vi "Read Rank.vi"(8 "error in":errorcluster, 11 "SA 26GHz Path Group in":refnum<class "SA 26GHz Path Group.lvclass">) -> (0 "error out":errorcluster, 2 "Rank":dbl, 3 "SA 26GHz Path Group out":refnum<class "SA 26GHz Path Group.lvclass">)   [LabVIEW 2023, in "RFFixtureCharact.PXI.lvlib" / "SA 26GHz Path Group.lvclass"]
uses:
  SA 26GHz Path Group.lvclass
  SA 26GHz Path Group.lvclass/SA 26GHz Path Group.ctl
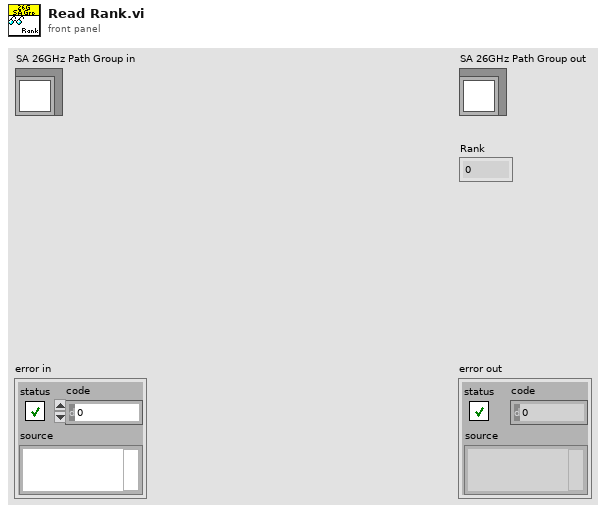
[diagram p1: front panel]
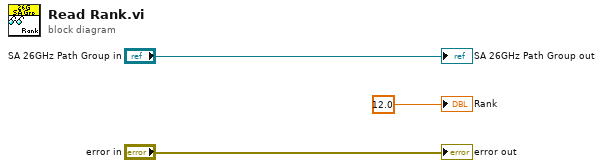
[diagram p0: block diagram]
diagram:
  "error out" <- "error in"
  "SA 26GHz Path Group out" <- "SA 26GHz Path Group in"
  "Rank" <- 12.0 ("Rank")
